vi "NanotecSMCPD.ID query.vi"(0 "i ref in":refnum<vi>, 3 "ms timeout (10000)":i32=10000, 5 "error in (no error)":errorcluster) -> (14 "i ref out":refnum<vi>, 15 "deviceID":string, 17 "timed out":bool, 19 "error out":errorcluster)   [LabVIEW 2014, in "NanotecSMCPD.lvlib"]
doc: "Queries the device IDs from all controllers."
uses:
  NanotecSMCPD.lvlib
  CSCore/CSSystem/CoreDefs/CoreDefs.error_type.ctl
  CSCore/CSSystem/CoreDefs/CoreDefs.error_severity.ctl
  CSCore/CSApplicationBaseClasses/MotorBase/MotorBase.lvlib
  CSCore/CSSystem/CoreLib/CoreLib.lvlib
  CSCore/CSApplicationBaseClasses/DeviceBase/DeviceBase.lvlib
  CSinstr.lib/NanotecSMCPD/NanotecSMCPDDriver.lvlib
  CSlibraries/UtilityLib/UtilityLib.lvlib
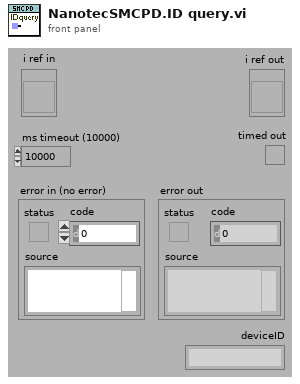
[diagram p1: front panel]
types:
  T1 = typedef "CoreDefs.error_severity.ctl" = enum16{"undefined", "information", "warning", "error", "fatal"}
  T2 = typedef "CoreDefs.error_type.ctl" = enum16{"no error", "can't load process", "can't unload process", "process does not exist", "can't install process", "can't remove process", "unknown function", "time out", "can't execute function", "duplicate queue name", "super not found", "caller queue invalid", "can't ping process", "unknown error", "VISA Error", "VISA timeout", "GPIB timeout", "GPIB error", "communication error", "data type mismatch", "can't read data from OPC server", "can't write data to OPC server", "OET error", "function not implemented", "process already exists", "invalid Shared Variable name", "error writing Shared Variable", "error reading Shared Variable", "invalid client name", "corrupt database", "unknown class", "call not authorized", "parameter out of range", "OET timeout: can't get data to modify", "invalid queue name", "requested operation incompatible with current state", "event undefined", "event disabled", "state undefined", "caller is not a friend", "EventBuilder: bad eventID", "EventBuilder: no DAQ devices", "a thread must not stop itself", "UNUSED ELEMENT4", "DiscArchiver: eventData incomplete", "DiscArchiver: eventData does not belong to run", "DiscArchiver: can't open file", "DiscArchiver: can't write to file", "DiscArchiver: available disc space low", "can't acquire semaphore", "error reading data from database", "notifier object is not existing", "can't register process", "can't unregister process", "illegal event type", "object disabled", "object already exists", "can't change state", "Instrument not found", "no connection to remote node", "invalid reference", "N/A", "UNUSED ELEMENT 1", "element not found", "illegal TCP/IP connection detected", "object does not exist", "invalid access ID", "unknown CS system", "invalid privilige", "unsupported data type", "unsupported server type", "IO server already exists", "Shared Variable already exists"}
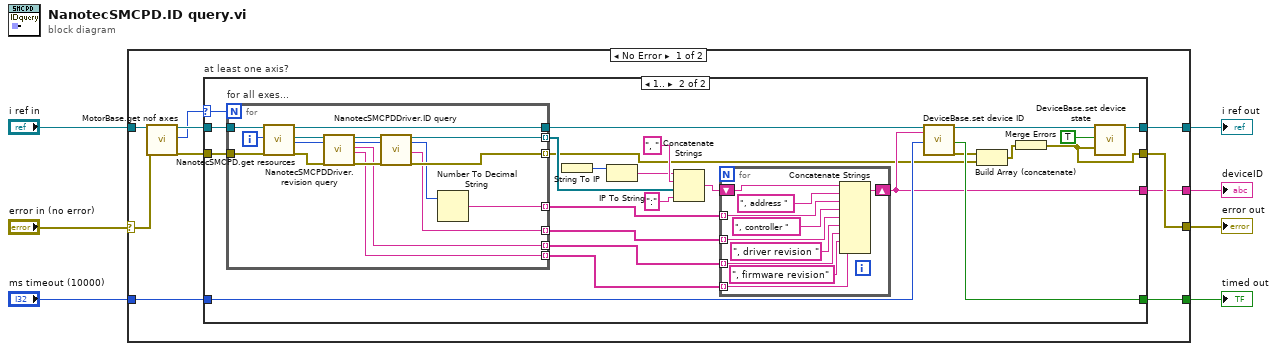
[diagram p0: block diagram]
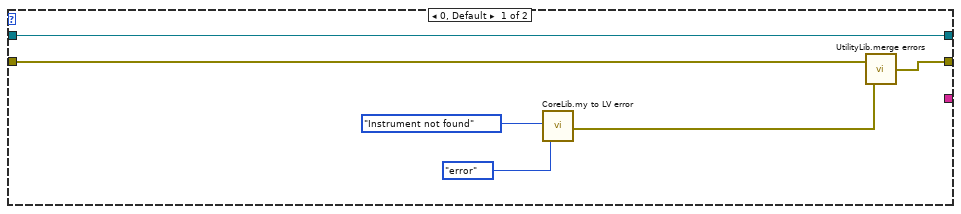
[diagram p2: hidden frame]
diagram:
  n1 = case shown="No Error" "error in (no error)" {
    selector: "error in (no error)" -> [w15 w75]
    tunnel: "i ref in" -> [w17 w76]
    tunnel: [w11 w76] -> w6
    tunnel: [w10 w75] -> w5
    tunnel: "ms timeout (10000)" -> [w14 _]
    tunnel: [w9 _] -> w2
    tunnel: [w8 _] -> w1
    frame No Error {
      n2 = call "MotorBase.get nof axes.vi"("i ref in"=w17, "error in (no error)"=w15) -> ("i ref out"=w16:refnum<vi>, "nOfAxis"=w12:i32, "error out"=w13:errorcluster)  [unwired: 15 in]
      n3 = case "at least one axis?" shown="1.." w12 {
        selector: w12 -> [_ w47]
        tunnel: w16 -> [w23 w46]
        tunnel: w14 -> [_ w43]
        tunnel: w13 -> [w19 w45]
        tunnel: [w23 w33] -> w11
        tunnel: [w18 w24] -> w10
        tunnel: [_ w42] -> w9
        tunnel: [_ w34] -> w8
        frame 0, Default {
          n4 = call "CoreLib.my to LV error.vi"("ErrorTypes"=CoreDefs.error_type."Instrument not found", "severityLevel"=CoreDefs.error_severity."error") -> ("myErrorCluster"=w20:errorcluster)  [unwired: 16 in, 1 out]
          n5 = call "UtilityLib.merge errors.vi"("error2 (no error)"=w20, "error1 (no error)"=w19) -> ("error out"=w18:errorcluster)
        }
        frame 1.. {
          n6 = for "for all exes..." {
            N: w47 -> [_]
            tunnel: w46 -> [w74]
            tunnel: [w70] -> w44
            tunnel: [w69] -> w38 mode=indexing
            tunnel: [w67] -> w36 mode=indexing
            tunnel: [w66] -> w30 mode=indexing
            tunnel: [w59] -> w29 mode=indexing
            tunnel: [w58] -> w28 mode=indexing
            tunnel: w45 -> [w73]
            tunnel: [w71] -> w26 mode=indexing
            i -> [w72]
            n7 = call "NanotecSMCPD.get resources.vi"("i ref in"=w74, "axisNumber"=w72, "error in (no error)"=w73) -> ("i ref out"=w70:refnum<vi>, "VISA resource"=w65:refnum<visa-resource-name>, "address"=w63:i32, "error out"=w61:errorcluster)  [unwired: 13 in]
            n8 = call "NanotecSMCPDDriver.revision query.vi"("VISA resource name"=w65, "contollerID"=w63, "error in (no error)"=w61) -> ("VISA resource name out"=w64:refnum<visa-resource-name>, "contollerID out"=w62:i32, "Instrument Driver Revision"=w59:string, "Instrument Firmware Revision"=w58:string, "error out"=w60:errorcluster)  [unwired: 12 in]
            n9 = call "NanotecSMCPDDriver.ID query.vi"("VISA resource name"=w64, "contollerID"=w62, "error in (no error)"=w60) -> ("VISA resource name out"=w69:refnum<visa-resource-name>, "contollerID out"=w68:i32, "hardwareTypeString"=w66:string, "error out"=w71:errorcluster)  [unwired: 12 in, 1 out]
            n10 = Number To Decimal String(number=w68) -> (decimal integer string=w67:string)  [unwired: 1 in]
          }
          n11 = String To IP() -> (0:w41:u32)  [unwired: 1 in]
          n12 = IP To String(2:w41) -> (0:w39:string)  [unwired: 1 in]
          n13 = Concatenate Strings(w39, ", " ("string"), w38, ":" ("string")) -> (w37:string)
          n14 = for {
            shift-right: [w57] -> w34
            shift-left: w37 -> [w56]
            tunnel: w36 -> [w55] mode=indexing
            tunnel: w30 -> [w54] mode=indexing
            tunnel: w29 -> [w53] mode=indexing
            tunnel: w28 -> [w48] mode=indexing
            n15 = Concatenate Strings(w56, ", address " ("string"), w55, ", controller " ("string"), w54, ", driver revision " ("string"), w53, ", firmware revision" ("string"), w48) -> (w57:string)
          }
          n16 = call "DeviceBase.set device ID.vi"("i ref in"=w44, "deviceID"=w34, "ms timeout (10000)"=w43) -> ("i ref out"=w32:refnum<vi>, "timed out"=w42:bool, "error out"=w27:errorcluster)  [unwired: 14 in]
          n17 = Build Array (concatenate)(w27, w26) -> (w25:errorcluster[])
          n18 = Merge Errors(w25) -> (w24:errorcluster)
          n19 = call "DeviceBase.set device state.vi"("i ref in"=w32, "implicit"=TRUE, "device error"=w24) -> ("i ref out"=w33:refnum<vi>)  [unwired: 14 in, 2 out]
        }
      }
    }
    frame Error {
    }
  }
  "error out" <- w5
  "i ref out" <- w6
  "timed out" <- w2
  "deviceID" <- w1
